vi "STAGE+mono+counter_edit6.vi"() -> ()   [LabVIEW 2017]
panel:
  out "Waveform Graph 2":waveform(dbl)(graph) caption="Record 41  of  100"
  out "Waveform Graph":waveform(dbl)(graph) caption="Record 41  of  100"
  in  "scan from 2":i32=2600
  in  "Integrating time, 10^-7 sec":dbl=10000000.0
  out "Timeout 2":bool
  in  "scan from":i32=2600
  in  "scan to":i32=4000
  in  "?":bool
  in  "Exit Labview":bool
  in  "step size":dbl=10.0 min=0.0
  in  "?":bool
  out "Counts":i32
  in  "value (0)":dbl=-9.0
  out "Current WL Wavelength  2":u16 caption="Current Wavelength"
  out "Grt# 2":u8=1 min=1 max=3 step=1
  out "Blaze (nm)":u32=300
  out "Groove/mm":u32=1200
  in  "?":bool
  in  "Channel B Input":u16(ring)=2 items=["Input 1"=1, "Input 2"=2]
  in  "Trigger mode":u16(ring) items=["10 MHz"=0, "Input 2"=2, "Input T"=3]
  out "Current WL Wavelength":u16 caption="Current Wavelength"
  in  "Integrating time, 10^-7 sec":dbl=10000000.0
  in  "gate A mode (CW:0)":i16(slide) scale=0.0..2.0 scale format="%.2f"
  in  "Channel A Input":u16(ring)=1 items=["10 MHz", "Input 1"]
  in  "Time between measurements\n at one point (s)/Dwell Time":dbl=0.002 min=0.002 max=60.0 step=0.001
  in  "Number of Measurements\n to take at one point/ Number of Periods":u16=1 min=1 max=2000 step=1
  in  "Count Mode":u16(ring) items=["A,B for Preset T", "A-B for Preset T", "A+B for Preset T", "A for Preset B"]
  in  "GPIB address":string="23"
  out "Timeout":bool
  out "Serial":u32=12345
  out "Grt#":u8=1 min=1 max=3 step=1
  out "Blaze (nm)":u32=300
  out "Groove/mm":u32=1200
  out "time delay":u32=450000 min=1
  out "Mono port":T1(ring)
  in  "Get position":bool
  out "Position status":dbl format="%.3f"
  in  "Target position":dbl format="%.3f"
  in  "Move":bool
  in  "Motor OFF":bool
  in  "Motor ON":bool
  in  "Step Size [um]":i32=10
  in  "Axis":i32=1
  in  "Rep Rate [Hz]":dbl=500.0
  out "Shots":dbl
  in  "Averaging Time [s]":dbl=0.1
  out "Current Point":i32
  out "Slide":i32(slide) scale=0.0..100.0
  out "Current Position [mm]":dbl
  in  "Axis initial position [mm]":dbl
  out "Axis final Position [mm]":dbl
  in  "Data Points (100 default)":i32=100
  in  "Collect Data!":bool
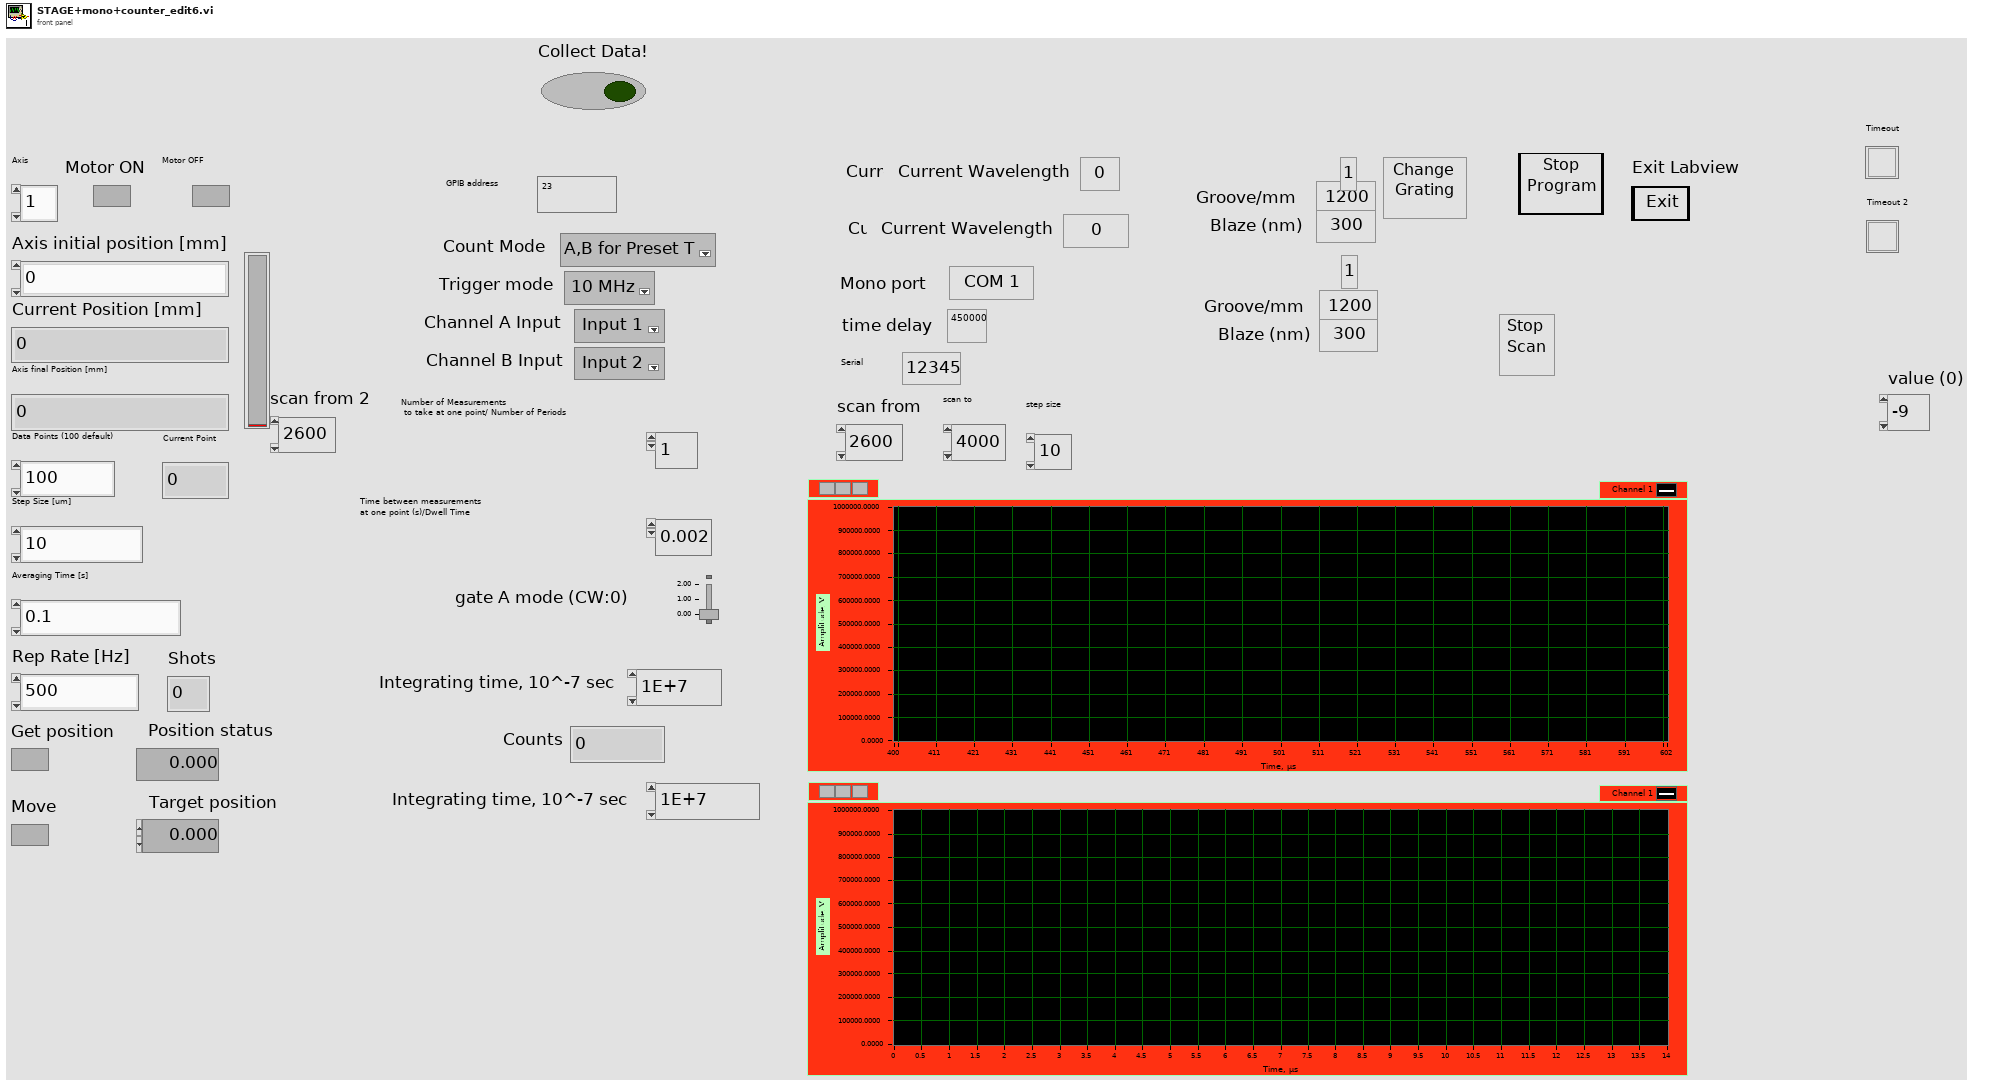
[diagram p1: front panel]
types:
  T1 = enum8{"COM 1", "COM 2", "COM 3", "COM 4", "COM 5", "COM 6", "COM 7", "COM 8", "COM 9"}
  T2 = cluster{"input XON/XOFF":bool, "input HW Handshake":bool, "input alt HW HShk":bool, "output XON/XOFF":bool, "output HW Handshake":bool, "output alt HW HShk":bool, "XOFF byte":u8, "XON byte":u8, "parity error byte":u16}
  T3 = enum16{"no parity", "odd parity", "even parity", "mark parity", "space parity"}
  T4 = cluster{"Y[0]":dbl, "Y[1]":dbl, "Y[2]":dbl, "Y[3]":dbl, "Y[4]":dbl, "Y[5]":dbl, "Y[6]":dbl, "Y[7]":dbl, "Y[8]":dbl}
  T5 = typedef "NI_Matrix.lvlib/RealMatrix.ctl" = dbl[][]
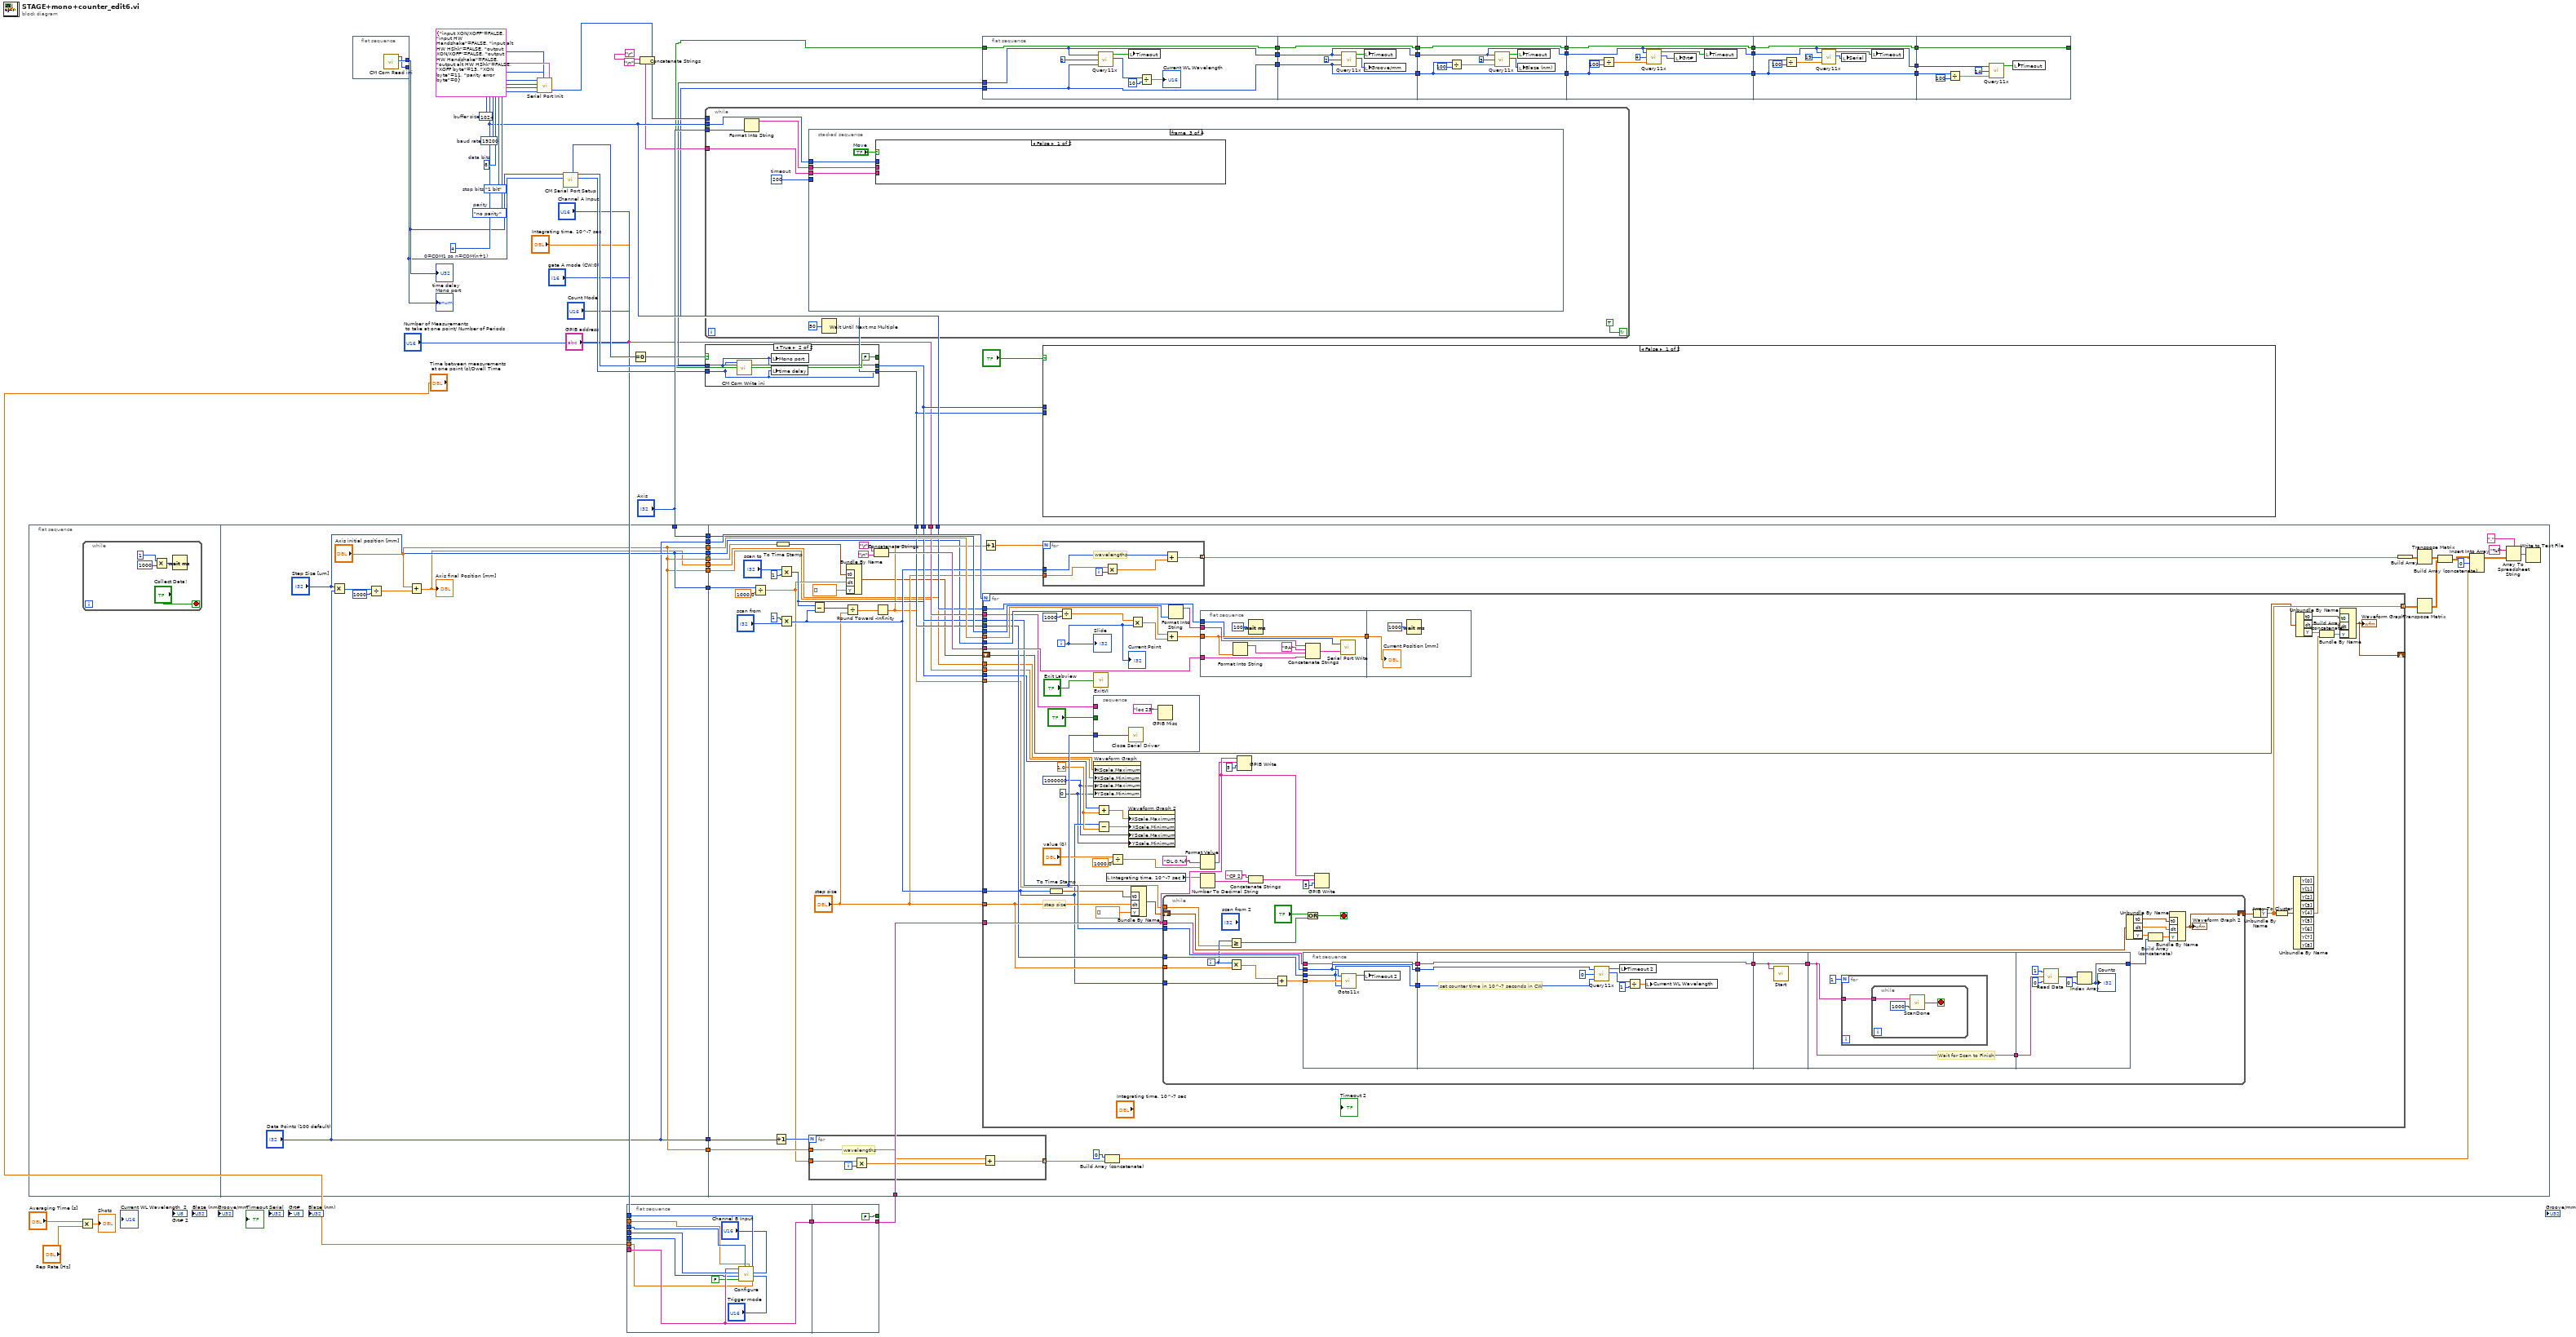
[diagram p0: block diagram]
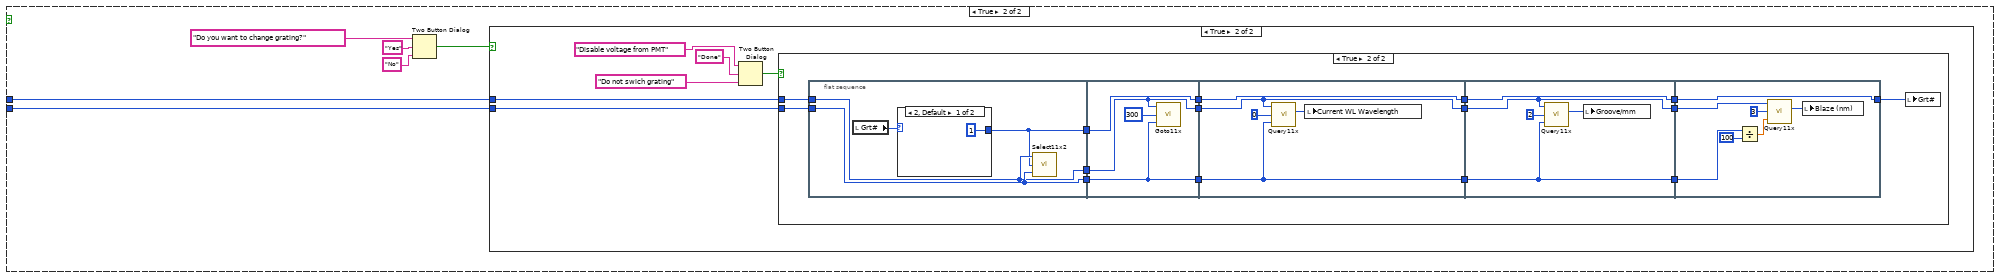
[diagram p2: hidden frame]
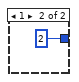
[diagram p5: hidden frame]
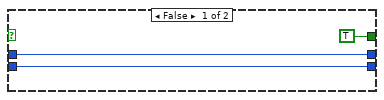
[diagram p6: hidden frame]
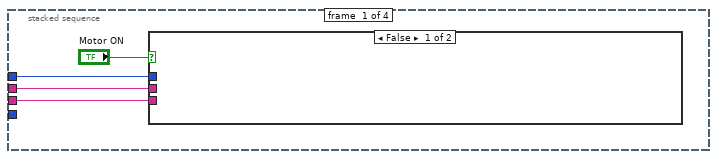
[diagram p7: hidden frame]
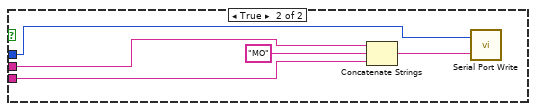
[diagram p8: hidden frame]
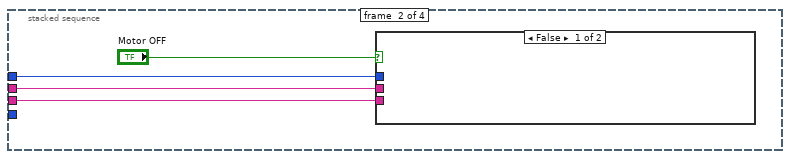
[diagram p9: hidden frame]
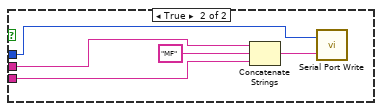
[diagram p10: hidden frame]
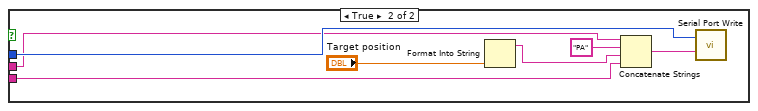
[diagram p11: hidden frame]
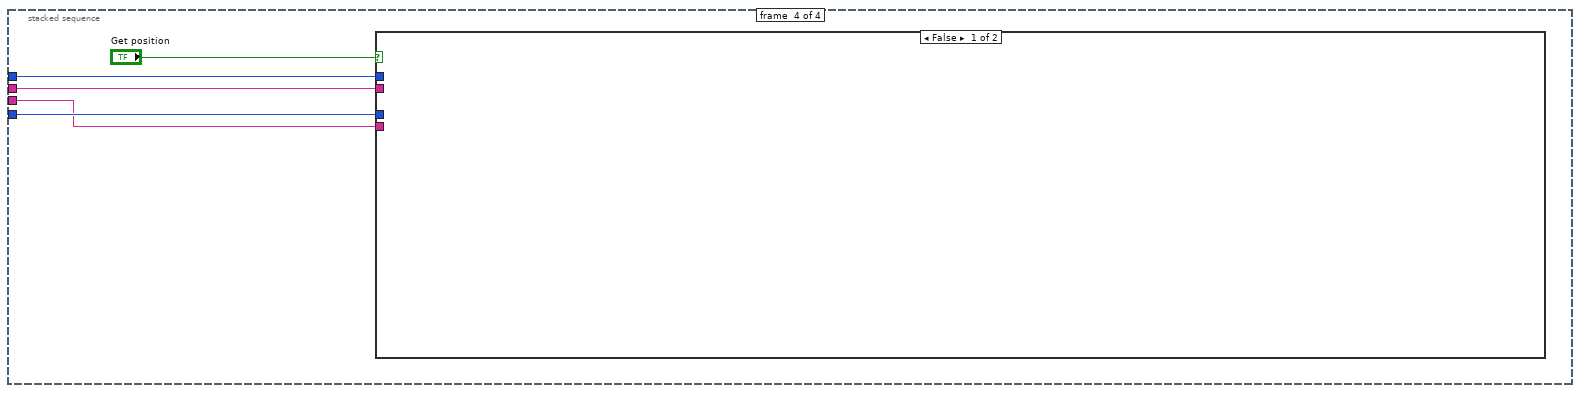
[diagram p12: hidden frame]
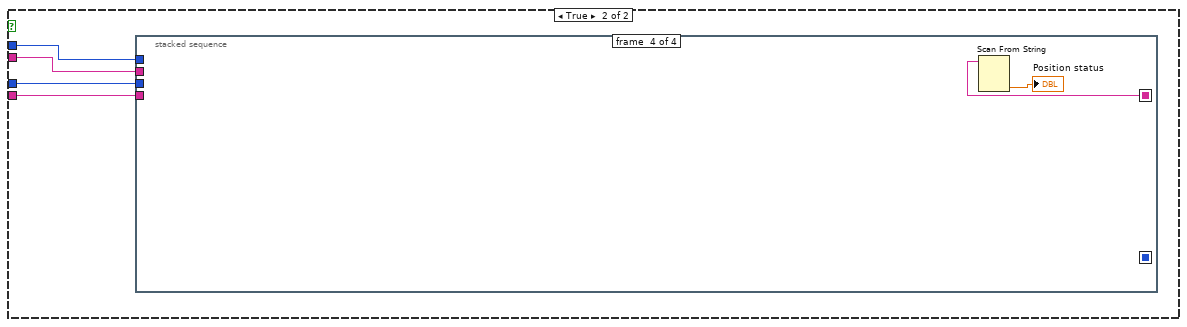
[diagram p13: hidden frame]
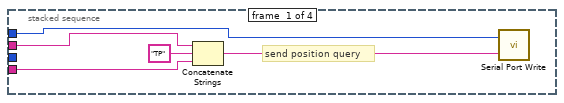
[diagram p14: hidden frame]
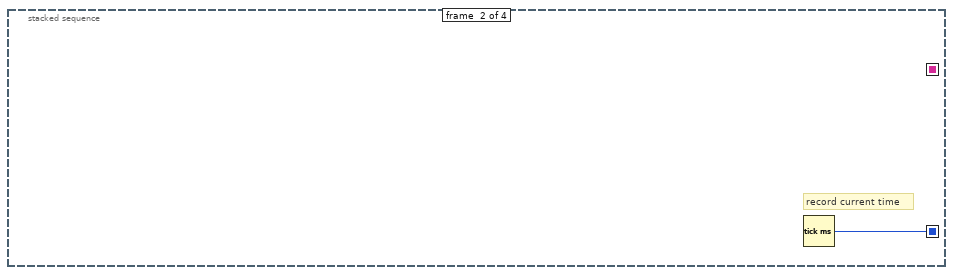
[diagram p15: hidden frame]
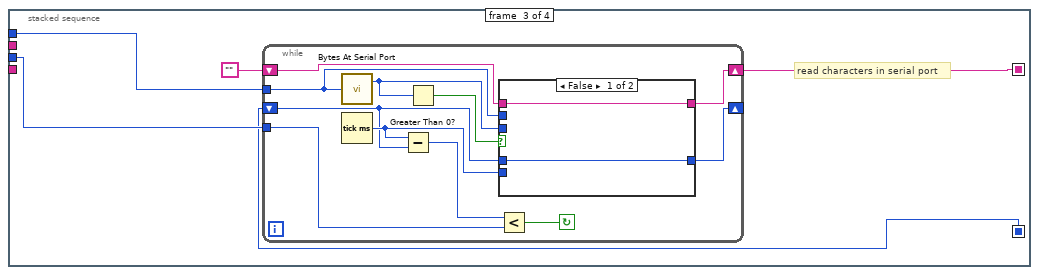
[diagram p16: hidden frame]
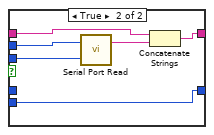
[diagram p17: hidden frame]
diagram:
  w50 = u32 19200  # baud rate
  w49 = u16 8  # data bits
  w48 = enum16{"1 bit", "1.5 bits", "2 bits"}."1 bit"  # stop bits
  w53 = T3."no parity"  # parity
  w47 = 4  # 0=COM1 so n=COM(n+1)
  w52 = u16 1024  # buffer size
  n1 = flat-sequence {
    tunnel: ["Data Points (100 default)"] -> w59
    tunnel: "Axis" -> [w71]
    tunnel: ["Axis initial position [mm]"] -> w58
    tunnel: [w71] -> w57
    tunnel: ["Axis initial position [mm]"] -> w7
    tunnel: ["Step Size [um]"] -> w6
    tunnel: ["Axis initial position [mm]"] -> w5
    tunnel: ["Step Size [um]"] -> w4
    tunnel: ["Data Points (100 default)"] -> w3
    tunnel: ["Axis initial position [mm]"] -> w2
    tunnel: [w64] -> w1
    tunnel: w59 -> [w120]
    tunnel: w58 -> [w119]
    tunnel: w57 -> [w118]
    tunnel: w47 -> [w114]
    tunnel: w11 -> [w113]
    tunnel: w10 -> [w112]
    tunnel: w9 -> [w111]
    tunnel: "GPIB address" -> [w110]
    tunnel: w7 -> [w90]
    tunnel: w6 -> [w89]
    tunnel: w5 -> [w83]
    tunnel: w4 -> [w82]
    tunnel: w3 -> [w80]
    tunnel: w2 -> [w73]
    tunnel: w1 -> [w72]
    frame #0 {
      n2 = while {
        stop <- "Collect Data!" stop-if-true
        n3 = Multiply(x=1, y=1000) -> (x*y=w63:i32)
        n4 = Wait (ms)(milliseconds to wait=w63) -> ()  [unwired: 1 out]
      }
    }
    frame #1 {
      n5 = Multiply(x="Step Size [um]", y="Data Points (100 default)") -> (x*y=w69:i32)
      n6 = Divide(x=w69, y=1000) -> (x/y=w68:dbl)
      n7 = Add(x="Axis initial position [mm]", y=w68) -> (x+y=w64:dbl)
      "Axis final Position [mm]" <- w64
    }
    frame #2 {
      n8 = Divide(x=w89, y=1000.0) -> (x/y=w81:dbl)
      n9 = Increment(x=w80) -> (x+1=w84:i32)
      n10 = To Time Stamp(1:w90) -> (0:w88:timestamp)
      n11 = Multiply(x="scan to", y=1) -> (x*y=w102:i32)
      n12 = Multiply(x=1, y="scan from") -> (x*y=w105:i32)
      n13 = for {
        N: w84 -> [_]
        tunnel: w81 -> [w125]
        tunnel: w83 -> [w123]
        tunnel: [w121] -> w78 mode=indexing
        i -> [w124]
        # "wavelengths"
        n14 = Multiply(x=w125, y=w124) -> (x*y=w122:dbl)
        n15 = Add(x=w123, y=w122) -> (x+y=w121:dbl)
      }
      n16 = Subtract(x=w102, y=w105) -> (x-y=w100:i32)
      n17 = Divide(x=w100, y="step size") -> (x/y=w99:dbl)
      n18 = Bundle By Name("t0"=w88, "dt"=w81, "Y"=dbl[] []) -> (w85:waveform(dbl))  [unwired: 1 in]
      n19 = Concatenate Strings("\r", "\n") -> (w115:string)
      n20 = Round Toward -Infinity(1:w99) -> (0:w98:dbl)
      n21 = for {
        N: w120 -> [_]
        tunnel: w119 -> [w183]
        tunnel: w82 -> [w179]
        tunnel: w118 -> [w176]
        tunnel: w115 -> [w173]
        tunnel: w114 -> [w174]
        tunnel: w113 -> [w171]
        tunnel: w112 -> [w168]
        tunnel: w111 -> [w170]
        tunnel: w110 -> [w169]
        tunnel: [w146] -> w93 mode=indexing
        tunnel: w105 -> [w135]
        tunnel: w102 -> [w151]
        tunnel: "step size" -> [w150]
        tunnel: w98 -> [w149]
        shift-right: [w138] -> _
        shift-left: w85 -> [w142]
        tunnel: w73 -> [w137]
        tunnel: w72 -> [w136]
        i -> [w148]
        w131 = 0
        w132 = 1000000
        w166 = 1.0 ("x")
        # "step size"
        n22 = To Time Stamp(1:w135) -> (0:w163:timestamp)
        n23 = Divide(x=w179, y=1000) -> (x/y=w178:dbl)
        n24 = call "ExitVI.vi"("Exit Labview"="Exit Labview") -> ()
        n25 = stacked-sequence {
          tunnel: "?" -> [_]
          tunnel: w168 -> [w236]
          tunnel: w169 -> [_]
          frame #0 {
            n26 = call <vilib>:"Close Serial Driver.vi"("port number"=w236) -> ()  [unwired: 1 out]
            n27 = GPIB Misc(0:"loc 23" ("command string")) -> ()  [unwired: 1 in, 3 out]
          }
        }
        n28 = property on="Waveform Graph" class="WFGraph (strict)"("XScale.Maximum"=w136, "XScale.Minimum"=w137, "YScale.Maximum"=w132, "YScale.Minimum"=w131) -> ()  [unwired: 2 in, 2 out]
        n29 = Add(x=w151, y=w166) -> (x+y=w134:dbl)
        n30 = Subtract(x=w135, y=w166) -> (x-y=w133:dbl)
        n31 = local read "Integrating time, 10^-7 sec"() -> (w165:dbl)
        n32 = Divide(x="value (0)", y=1000.0) -> (x/y=w152:dbl)
        n33 = property on="Waveform Graph 2" class="WFGraph (strict)"("XScale.Maximum"=w134, "XScale.Minimum"=w133, "YScale.Maximum"=w132, "YScale.Minimum"=w131) -> ()  [unwired: 2 in, 2 out]
        n34 = Multiply(x=w178, y=w148) -> (x*y=w182:dbl)
        n35 = Bundle By Name("t0"=w163, "dt"=w150, "Y"=dbl[] []) -> (w162:waveform(dbl))  [unwired: 1 in]
        n36 = while {
          tunnel: w168 -> [w207]
          tunnel: w170 -> [w206]
          shift-right: [w184] -> w157
          shift-left: w162 -> [w204]
          tunnel: w171 -> [w196]
          tunnel: w135 -> [w187]
          tunnel: w150 -> [w186]
          tunnel: w149 -> [w185]
          i -> [w201]
          stop <- w205 stop-if-true
          n37 = Greater Or Equal?(x=w201, y=w185) -> (x >= y?=w197:bool)
          n38 = Multiply(x=w201, y=w186) -> (x*y=w208:dbl)
          n39 = Add(x=w208, y=w187) -> (x+y=w188:dbl)
          n40 = flat-sequence {
            tunnel: w188 -> [w213]
            tunnel: w207 -> [w212]
            tunnel: [w212] -> w194
            tunnel: w206 -> [w211]
            tunnel: [w211] -> w193
            tunnel: w196 -> [w209]
            tunnel: [w209] -> w192
            tunnel: w194 -> [w220]
            tunnel: w193 -> [w219]
            tunnel: w192 -> [w217]
            tunnel: [w217] -> w191
            tunnel: w191 -> [w222]
            tunnel: [w222] -> w190
            tunnel: w190 -> [w223]
            tunnel: [w223] -> w189
            tunnel: w189 -> [w230]
            tunnel: [w229] -> w195
            frame #0 {
              n41 = call "Goto11x.vi"("time delay"=w211, "WAVELENGTH"=w213, "port number"=w212) -> ("timeout"=w210:bool)  [unwired: 2 out]
              n42 = local write "Timeout 2"(w210) -> ()
            }
            frame #1 {
              # "set counter time in 10^-7 seconds in CW"
              n43 = call "Query11x.vi"("port number"=w220, "QUERY"=0, "time delay"=w219) -> ("timeout"=w218:bool, "STATUS MESSAGE"=w216:u16)  [unwired: 2 out]
              n44 = local write "Timeout 2"(w218) -> ()
              n45 = Divide(x=w216, y=1) -> (x/y=w215:dbl)
              n46 = local write "Current WL Wavelength"(w215) -> ()
            }
            frame #2 {
              n47 = call "Start.vi"("GPIB Address"=w222) -> ()  [unwired: 9 in]
            }
            frame #3 {
              # "Wait for Scan to Finish"
              n48 = for {
                N: 1 -> [_]
                tunnel: w223 -> [w225]
                n49 = while {
                  tunnel: w225 -> [w226]
                  stop <- w228 stop-if-true
                  n50 = call "ScanDone.vi"("Wait (ms)"=1000, "GPIB Address"=w226) -> ("Scan Finished?"=w228:bool)
                }
              }
            }
            frame #4 {
              n51 = call "Read Data.vi"("Channel Number"=0, "GPIB Address"=w230, "Number of Datapoints"=1) -> ("Data"=w231:i32[])
              n52 = Index Array(array=w231, index=0) -> (element=w229:i32)
              "Counts" <- w229
            }
          }
          n53 = Or(x="?", y=w197) -> (x .or. y?=w205:bool)
          n54 = Unbundle By Name(w204) -> ("t0"=w202:timestamp, "dt"=w203:dbl, "Y"=w200:dbl[])
          n55 = Build Array (concatenate)(w200, w195) -> (w199:dbl[])
          n56 = Bundle By Name("t0"=w202, "dt"=w203, "Y"=w199) -> (w184:waveform(dbl))  [unwired: 1 in]
          "Waveform Graph 2" <- w184
        }
        n57 = Add(x=w183, y=w182) -> (x+y=w181:dbl)
        n58 = Format Into String(w176) -> (resulting string=w175:string)  [unwired: 3 in, 1 out]
        n59 = flat-sequence {
          tunnel: w181 -> [w239]
          tunnel: [w239] -> w177
          tunnel: w173 -> [w241]
          tunnel: w175 -> [w240]
          tunnel: w174 -> [w237]
          tunnel: w177 -> [w245]
          frame #0 {
            n60 = Format Into String(w239) -> (resulting string=w238:string)  [unwired: 3 in, 1 out]
            n61 = Wait (ms)(milliseconds to wait=u32 100) -> ()  [unwired: 1 out]
            n62 = Concatenate Strings(w240, "PA" ("Substring"), w238, w241) -> (w243:string)
            n63 = call <vilib>:"Serial Port Write.vi"("string to write"=w243, "port number"=w237) -> ()  [unwired: 1 out]
          }
          frame #1 {
            n64 = Wait (ms)(milliseconds to wait=u32 1000) -> ()  [unwired: 1 out]
            "Current Position [mm]" <- w245
          }
        }
        n65 = Format Value(format string="DL 0,%f;", value (0)=w152) -> (output string=w155:string)  [unwired: 1 in]
        n66 = Number To Decimal String(number=w165) -> (decimal integer string=w160:string)  [unwired: 1 in]
        n67 = GPIB Write(0:w171, 1:w155, 2:i16 5 ("mode (0)")) -> ()  [unwired: 2 in, 2 out]
        n68 = Concatenate Strings("CP 2,", w160) -> (w158:string)
        n69 = GPIB Write(0:w171, 1:w158, 2:i16 5 ("mode (0)")) -> ()  [unwired: 2 in, 2 out]
        n70 = Unbundle By Name(w157) -> ("Y"=w146:dbl[])
        n71 = Array To Cluster(array=w146) -> (cluster=w145:T4)
        n72 = Unbundle By Name(w145) -> ("Y[4]"=w141:dbl)  [unwired: 8 out]
        n73 = Unbundle By Name(w142) -> ("t0"=w144:timestamp, "dt"=w143:dbl, "Y"=w140:dbl[])
        n74 = Build Array (concatenate)(w140, w141) -> (w139:dbl[])
        n75 = Bundle By Name("t0"=w144, "dt"=w143, "Y"=w139) -> (w138:waveform(dbl))  [unwired: 1 in]
        "Waveform Graph" <- w138
        "Current Point" <- w148
        "Slide" <- w148
      }
      n76 = Increment(x=w98) -> (x+1=w97:dbl)
      n77 = for {
        N: w97 -> [_]
        tunnel: "step size" -> [w130]
        tunnel: w105 -> [w128]
        tunnel: [w126] -> w95 mode=indexing
        i -> [w129]
        # "wavelengths"
        n78 = Multiply(x=w130, y=w129) -> (x*y=w127:dbl)
        n79 = Add(x=w128, y=w127) -> (x+y=w126:dbl)
      }
      n80 = Build Array (concatenate)(0, w78) -> (w77:dbl[])
      n81 = Build Array(w95) -> (w94:dbl[][])
      n82 = Transpose Matrix(1:w94) -> (0:w92:dbl[][])
      n83 = Transpose Matrix(1:w93) -> (0:w91:dbl[][])
      n84 = Build Array (concatenate)(w92, w91) -> (w75:T5)
      n85 = Insert Into Array(array=w75, index (row)=0, new element=w77) -> (w74:T5)  [unwired: 1 in]
      n86 = Array To Spreadsheet String(delimiter (Tab)=",", array=w74, 3:"%f" ("format string")) -> (spreadsheet string=w96:string)
      n87 = Write to Text File(text=w96) -> ()  [unwired: 3 in, 3 out]
    }
  }
  n88 = Multiply(x="Averaging Time [s]", y="Rep Rate [Hz]") -> (x*y=→"Shots":dbl)
  n89 = flat-sequence {
    tunnel: [w248] -> w25
    tunnel: [w247] -> w24
    frame #0 {
      n90 = call "CM Com Read ini.vi"() -> ("Mono port"=w247:T1, "time delay1"=w248:u32)  [unwired: 7 in]
    }
  }
  n91 = call <vilib>:"Serial Port Init.vi"("flow control etc."=T2 {"input XON/XOFF"=FALSE, "input HW Handshake"=FALSE, "input alt HW HShk"=FALSE, "output XON/XOFF"=FALSE, "output HW Handshake"=FALSE, "output alt HW HShk"=FALSE, "XOFF byte"=13, "XON byte"=11, "parity error byte"=0}, "parity"=w53, "buffer size"=w52, "stop bits"=w48, "data bits"=w49, "baud rate"=w50, "port number"=w47) -> ("error code"=w46:i32)
  n92 = call "CM Serial Port Setup.vi"("COM port"=w24, "time delay"=w25) -> ("time delay1"=w20:u32, "DK port Out"=w21:T1, "error code"=w23:i32)  [unwired: 7 in]
  n93 = flat-sequence {
    tunnel: "GPIB address" -> [w256]
    tunnel: [w256] -> w26
    tunnel: "Count Mode" -> [w257]
    tunnel: "Number of Measurements\n to take at one point/ Number of Periods" -> [w254]
    tunnel: "Time between measurements\n at one point (s)/Dwell Time" -> [w253]
    tunnel: "Channel A Input" -> [w258]
    tunnel: "gate A mode (CW:0)" -> [w250]
    tunnel: "Integrating time, 10^-7 sec" -> [w249]
    tunnel: w26 -> [w259]
    tunnel: [w259] -> w11
    tunnel: [FALSE] -> _
    frame #0 {
      n94 = call "Configure.vi"("Dwell Time (s)"=w253, "Channel T Input"="Trigger mode", "Channel B Input"="Channel B Input", "Channel A Input"=w258, "Integrating time, 10^-7 sec"=w249, "gate mode (CW:0)"=w250, "Scan End Mode"=FALSE, "Number of Periods"=w254, "Count Mode"=w257, "GPIB Address"=w256) -> ()
    }
    frame #1 {
    }
  }
  n95 = Equal To 0?(x=w23) -> (x = 0?=w22:bool)
  n96 = Concatenate Strings("\r", "\n") -> (w42:string)
  n97 = while {
    tunnel: w47 -> [w263]
    tunnel: w42 -> [w264]
    tunnel: w46 -> [_]
    tunnel: "Axis" -> [w261]
    stop <- TRUE continue-if-true
    w262 = u32 200  # timeout
    n98 = Format Into String(w261) -> (resulting string=w265:string)  [unwired: 3 in, 1 out]
    n99 = stacked-sequence {
      tunnel: w265 -> [w269 w279 w288 w300]
      tunnel: w264 -> [w268 w278 w287 w297]
      tunnel: w263 -> [w270 w280 w289 w299]
      tunnel: w262 -> [_ _ _ w298]
      frame #0 {
        n100 = case shown="False" "Motor ON" {
          tunnel: w270 -> [_ w276]
          tunnel: w269 -> [_ w273]
          tunnel: w268 -> [_ w272]
          frame False {
          }
          frame True {
            n101 = Concatenate Strings(w273, "MO" ("Substring"), w272) -> (w274:string)
            n102 = call <vilib>:"Serial Port Write.vi"("string to write"=w274, "port number"=w276) -> ()  [unwired: 1 out]
          }
        }
      }
      frame #1 {
        n103 = case shown="False" "Motor OFF" {
          tunnel: w280 -> [_ w285]
          tunnel: w279 -> [_ w282]
          tunnel: w278 -> [_ w281]
          frame False {
          }
          frame True {
            n104 = Concatenate Strings(w282, "MF" ("Substring"), w281) -> (w283:string)
            n105 = call <vilib>:"Serial Port Write.vi"("string to write"=w283, "port number"=w285) -> ()  [unwired: 1 out]
          }
        }
      }
      frame #2 {
        n106 = case shown="False" "Move" {
          tunnel: w289 -> [_ w296]
          tunnel: w288 -> [_ w293]
          tunnel: w287 -> [_ w292]
          frame False {
          }
          frame True {
            n107 = Format Into String("Target position") -> (resulting string=w290:string)  [unwired: 3 in, 1 out]
            n108 = Concatenate Strings(w293, "PA" ("Substring"), w290, w292) -> (w294:string)
            n109 = call <vilib>:"Serial Port Write.vi"("string to write"=w294, "port number"=w296) -> ()  [unwired: 1 out]
          }
        }
      }
      frame #3 {
        n110 = case shown="False" "Get position" {
          tunnel: w300 -> [_ w305]
          tunnel: w299 -> [_ w304]
          tunnel: w298 -> [_ w303]
          tunnel: w297 -> [_ w302]
          frame False {
          }
          frame True {
            n111 = stacked-sequence {
              seq-local: [_ w311 _ _] -> [_ _ w313 _]
              seq-local: [_ _ w312 _] -> [_ _ _ w337]
              tunnel: w305 -> [w308 _ _ _]
              tunnel: w304 -> [w307 _ w316 _]
              tunnel: w303 -> [_ _ w314 _]
              tunnel: w302 -> [w306 _ _ _]
              frame #0 {
                # "send position query"
                n112 = Concatenate Strings(w308, "TP" ("Substring"), w306) -> (w309:string)
                n113 = call <vilib>:"Serial Port Write.vi"("string to write"=w309, "port number"=w307) -> ()  [unwired: 1 out]
              }
              frame #1 {
                # "record current time"
                n114 = Tick Count (ms)() -> (millisecond timer value=w311:u32)
              }
              frame #2 {
                # "read characters in serial port"
                n115 = while {
                  shift-left: w313 -> [w317]
                  shift-right: [w318] -> _
                  tunnel: w314 -> [w321]
                  shift-left: "" -> [w324]
                  shift-right: [w323] -> w312
                  tunnel: w316 -> [w325]
                  stop <- w320 continue-if-true
                  n116 = call <vilib>:"Bytes At Serial Port.vi"("port number"=w325) -> ("byte count"=w326:u32)  [unwired: 1 out]
                  n117 = Tick Count (ms)() -> (millisecond timer value=w319:u32)
                  n118 = Subtract(x=w319, y=w317) -> (x-y=w322:u32)
                  n119 = Greater Than 0?(x=w326) -> (x > 0?=w327:bool)
                  n120 = case shown="False" w327 {
                    tunnel: w326 -> [_ w335]
                    tunnel: w325 -> [_ w334]
                    tunnel: w324 -> [w329 w332]
                    tunnel: [w329 w331] -> w323
                    tunnel: [w328 w330] -> w318
                    tunnel: w319 -> [_ w330]
                    tunnel: w317 -> [w328 _]
                    frame False {
                    }
                    frame True {
                      n121 = call <vilib>:"Serial Port Read.vi"("requested byte count"=w335, "port number"=w334) -> ("string read"=w333:string)  [unwired: 1 out]
                      n122 = Concatenate Strings(w332, w333) -> (w331:string)
                    }
                  }
                  n123 = Less?(x=w322, y=w321) -> (x < y?=w320:bool)
                }
              }
              frame #3 {
                n124 = Scan From String(input string=w337) -> (output 1=→"Position status":dbl)  [unwired: 4 in, 3 out]
              }
            }
          }
        }
      }
    }
    n125 = Wait Until Next ms Multiple(millisecond multiple=u32 50) -> ()  [unwired: 1 out]
  }
  n126 = case shown="True" w22 {
    tunnel: w21 -> [w340 w343]
    tunnel: w20 -> [w339 w342]
    tunnel: [w340 w343] -> w10
    tunnel: [w339 w342] -> w9
    tunnel: [TRUE FALSE] -> w19
    frame False {
    }
    frame True {
      n127 = call "CM Com Write ini.vi"("time delay1"=w343, "Mono port"=w342) -> ()  [unwired: 7 in]
      n128 = local write "Mono port"(w343) -> ()
      n129 = local write "time delay"(w342) -> ()
    }
  }
  n130 = flat-sequence {
    tunnel: w9 -> [w349]
    tunnel: [w349] -> w41
    tunnel: w10 -> [w351]
    tunnel: [w351] -> w40
    tunnel: w19 -> [w347]
    tunnel: [w347] -> w39
    tunnel: w41 -> [w354]
    tunnel: [w354] -> w38
    tunnel: w40 -> [w356]
    tunnel: [w356] -> w37
    tunnel: w39 -> [w352]
    tunnel: [w352] -> w36
    tunnel: w38 -> [w364]
    tunnel: [w364] -> w35
    tunnel: w37 -> [w361]
    tunnel: [w361] -> w34
    tunnel: w36 -> [w358]
    tunnel: [w358] -> w33
    tunnel: w35 -> [w372]
    tunnel: [w372] -> w32
    tunnel: w34 -> [w369]
    tunnel: [w369] -> w31
    tunnel: w33 -> [w366]
    tunnel: [w366] -> w30
    tunnel: w32 -> [w380]
    tunnel: [w380] -> w29
    tunnel: w31 -> [w377]
    tunnel: [w377] -> w28
    tunnel: w30 -> [w374]
    tunnel: [w374] -> w27
    tunnel: w29 -> [w387]
    tunnel: w28 -> [w384]
    tunnel: [w382] -> _
    tunnel: w27 -> [w382]
    frame #0 {
      n131 = call "Query11x.vi"("port number"=w351, "QUERY"=u16 0, "time delay"=w349) -> ("timeout"=w348:bool, "STATUS MESSAGE"=w346:u16)  [unwired: 2 out]
      n132 = local write "Timeout"(w348) -> ()
      n133 = Divide(x=w346, y=10 ("Numeric")) -> (x/y=→"Current WL Wavelength":dbl)
    }
    frame #1 {
      n134 = call "Query11x.vi"("port number"=w356, "QUERY"=u16 2, "time delay"=w354) -> ("timeout"=w353:bool, "STATUS MESSAGE"=w355:u16)  [unwired: 2 out]
      n135 = local write "Timeout"(w353) -> ()
      n136 = local write "Groove/mm"(w355) -> ()
    }
    frame #2 {
      n137 = Divide(x=w364, y=i16 100 ("device (1)")) -> (x/y=w362:dbl)
      n138 = call "Query11x.vi"("port number"=w361, "QUERY"=u16 3, "time delay"=w362) -> ("timeout"=w359:bool, "STATUS MESSAGE"=w360:u16)  [unwired: 2 out]
      n139 = local write "Timeout"(w359) -> ()
      n140 = local write "Blaze (nm)"(w360) -> ()
    }
    frame #3 {
      n141 = Divide(x=w372, y=i16 100 ("device (1)")) -> (x/y=w370:dbl)
      n142 = call "Query11x.vi"("port number"=w369, "QUERY"=u16 4, "time delay"=w370) -> ("timeout"=w367:bool, "STATUS MESSAGE"=w368:u16)  [unwired: 2 out]
      n143 = local write "Grt#"(w368) -> ()
      n144 = local write "Timeout"(w367) -> ()
    }
    frame #4 {
      n145 = Divide(x=w380, y=i16 100 ("device (1)")) -> (x/y=w378:dbl)
      n146 = call "Query11x.vi"("port number"=w377, "QUERY"=u16 19, "time delay"=w378) -> ("timeout"=w375:bool, "STATUS MESSAGE"=w376:u16)  [unwired: 2 out]
      n147 = local write "Serial"(w376) -> ()
      n148 = local write "Timeout"(w375) -> ()
    }
    frame #5 {
      n149 = Divide(x=w387, y=i16 100 ("device (1)")) -> (x/y=w385:dbl)
      n150 = call "Query11x.vi"("port number"=w384, "QUERY"=u16 14, "time delay"=w385) -> ("timeout"=w383:bool)  [unwired: 3 out]
      n151 = local write "Timeout"(w383) -> ()
    }
  }
  n152 = case shown="False" "?" {
    tunnel: w9 -> [_ w390]
    tunnel: w10 -> [_ w389]
    frame False {
    }
    frame True {
      n153 = Two Button Dialog(message="Do you want to change grating?", 1:"No" ("F button name (\"Cancel\")"), 2:"Yes" ("T button name (\"OK\")")) -> (T button?=w391:bool)
      n154 = case shown="True" w391 {
        tunnel: w390 -> [_ w396]
        tunnel: w389 -> [_ w395]
        frame False {
        }
        frame True {
          n155 = Two Button Dialog(message="Disable voltage from PMT", 1:"Do not swich grating" ("F button name (\"Cancel\")"), 2:"Done" ("T button name (\"OK\")")) -> (T button?=w397:bool)
          n156 = case shown="True" w397 {
            tunnel: w396 -> [_ w415]
            tunnel: w395 -> [_ w414]
            frame False {
            }
            frame True {
              n157 = flat-sequence {
                tunnel: w415 -> [w419]
                tunnel: [w419] -> w412
                tunnel: w414 -> [w418]
                tunnel: [w418] -> w411
                tunnel: [w416] -> w410
                tunnel: w412 -> [w423]
                tunnel: [w423] -> w409
                tunnel: w411 -> [w424]
                tunnel: [w424] -> w408
                tunnel: w410 -> [w422]
                tunnel: [w422] -> w407
                tunnel: w409 -> [w430]
                tunnel: [w430] -> w406
                tunnel: w408 -> [w429]
                tunnel: [w429] -> w405
                tunnel: w407 -> [w426]
                tunnel: [w426] -> w404
                tunnel: w406 -> [w433]
                tunnel: [w433] -> w403
                tunnel: w405 -> [w434]
                tunnel: [w434] -> w402
                tunnel: w404 -> [w431]
                tunnel: [w431] -> w401
                tunnel: w403 -> [w438]
                tunnel: w402 -> [w439]
                tunnel: [w436] -> w413
                tunnel: w401 -> [w436]
                frame #0 {
                  n158 = local read "Grt#"() -> (w417:u8)
                  n159 = case shown="2, Default" w417 {
                    tunnel: [1 2] -> w416
                    frame 2, Default {
                    }
                    frame 1 {
                    }
                  }
                  n160 = call "Select11x2.vi"("time delay"=w419, "NEW GRT?"=w416, "port number"=w418) -> ()  [unwired: 3 out]
                }
                frame #1 {
                  n161 = call "Goto11x.vi"("time delay"=w423, "WAVELENGTH"=u16 300, "port number"=w424) -> ()  [unwired: 3 out]
                }
                frame #2 {
                  n162 = call "Query11x.vi"("port number"=w429, "QUERY"=u16 0, "time delay"=w430) -> ("STATUS MESSAGE"=w427:u16)  [unwired: 3 out]
                  n163 = local write "Current WL Wavelength"(w427) -> ()
                }
                frame #3 {
                  n164 = call "Query11x.vi"("port number"=w434, "QUERY"=u16 2, "time delay"=w433) -> ("STATUS MESSAGE"=w432:u16)  [unwired: 3 out]
                  n165 = local write "Groove/mm"(w432) -> ()
                }
                frame #4 {
                  n166 = Divide(x=w438, y=i16 100 ("device (1)")) -> (x/y=w440:dbl)
                  n167 = call "Query11x.vi"("port number"=w439, "QUERY"=u16 3, "time delay"=w440) -> ("STATUS MESSAGE"=w437:u16)  [unwired: 3 out]
                  n168 = local write "Blaze (nm)"(w437) -> ()
                }
              }
              n169 = local write "Grt#"(w413) -> ()
            }
          }
        }
      }
    }
  }
  "Mono port" <- w24
  "time delay" <- w25
